vi "projection profile (SubVI).vi"(10 "r":dbl, 11 "input frame":u16[][](array[numeric])) -> (3 "Array":u32[](array[numeric]))   [LabVIEW 2024]
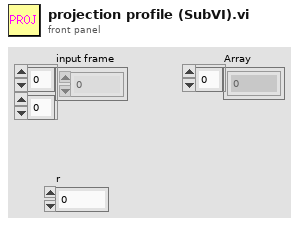
[diagram p1: front panel]
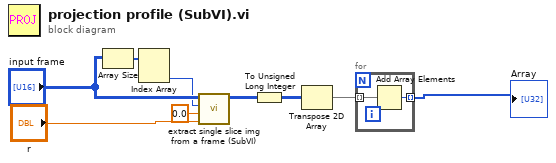
[diagram p0: block diagram]
diagram:
  n1 = Array Size(array="input frame") -> (size(s)=w2:i32[])
  n2 = Index Array(array=w2) -> (element #2=w1:i32)  [unwired: 2 in, 1 out]
  n3 = call "extract single slice img from a frame (SubVI).vi"("AOD scan speed ratio"="r", "init pos"=0.0, "Nx"=w1, "image in"="input frame") -> ("Array"=w8:u16[][])  [unwired: 7 in]
  n4 = To Unsigned Long Integer(number=w8) -> (unsigned 32bit integer=w7:u32[][])
  n5 = Transpose 2D Array(2D array=w7) -> (transposed array=w6:u32[][])
  n6 = for {
    tunnel: w6 -> [w11] mode=indexing
    tunnel: [w10] -> w5 mode=indexing
    n7 = Add Array Elements(numeric array=w11) -> (sum=w10:u32)
  }
  "Array" <- w5
